vi "Write Cipher.vi"(10 "Cipher":refnum<class "Cipher.lvclass">, 11 "Message Stream in":refnum<class "Message Stream.lvclass">) -> (3 "Message Stream out":refnum<class "Message Stream.lvclass">)   [LabVIEW 2020, in "Message Stream.lvclass"]
doc: "Use this accessor to specify the cipher that will be used to encrypt/decrypt messages exchanged by this stream. If no cipher is specified, messages will be exchanged in plaintext."
uses:
  Message Stream.lvclass
  Cipher/Cipher.lvclass
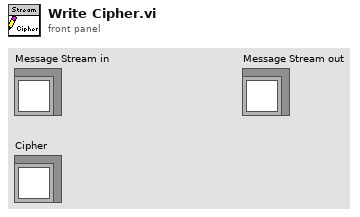
[diagram p1: front panel]
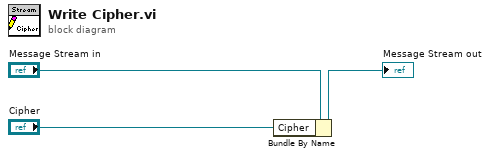
[diagram p0: block diagram]
diagram:
  n1 = Bundle By Name(cluster="Message Stream in", "Cipher"="Cipher") -> (→"Message Stream out":refnum<class "Message Stream.lvclass">)
